vi "DAQ-AI Mean Value.vi"(8 "Cluster":T1, 11 "data":dbl[][](array[numeric]) format="%0.2f") -> (3 "Analoge Input":dbl[](array[numeric]))   [LabVIEW 2015]
uses:
  <vilib>/Analysis/baseanly.llb/Mean (DBL).vi
  Galobal variable_TI.vi
  <vilib>/Analysis/NI_AALBase.lvlib
  <vilib>/ptbypt/NI_PtbyPt.lvlib
panel:
  out "AI_as DI":bool[](array[boolean])
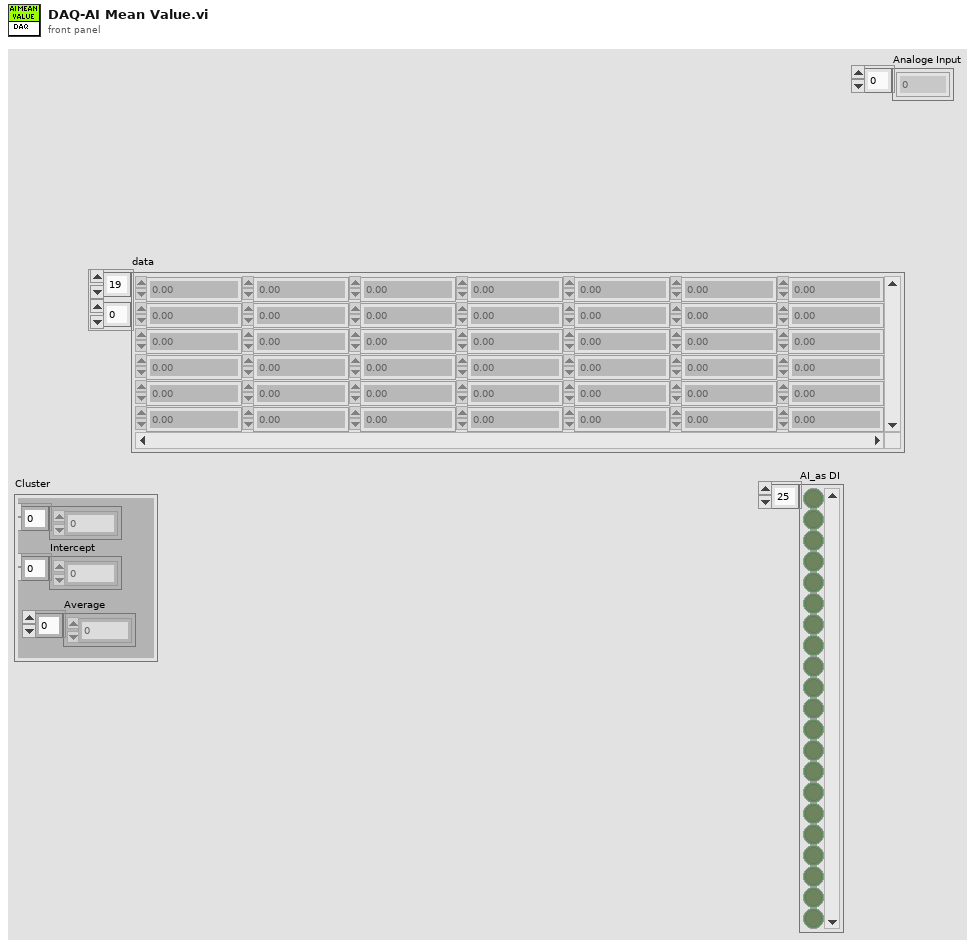
[diagram p1: front panel]
types:
  T1 = cluster{"Slop":dbl[], "Intercept":dbl[], "Average ":i16[]}
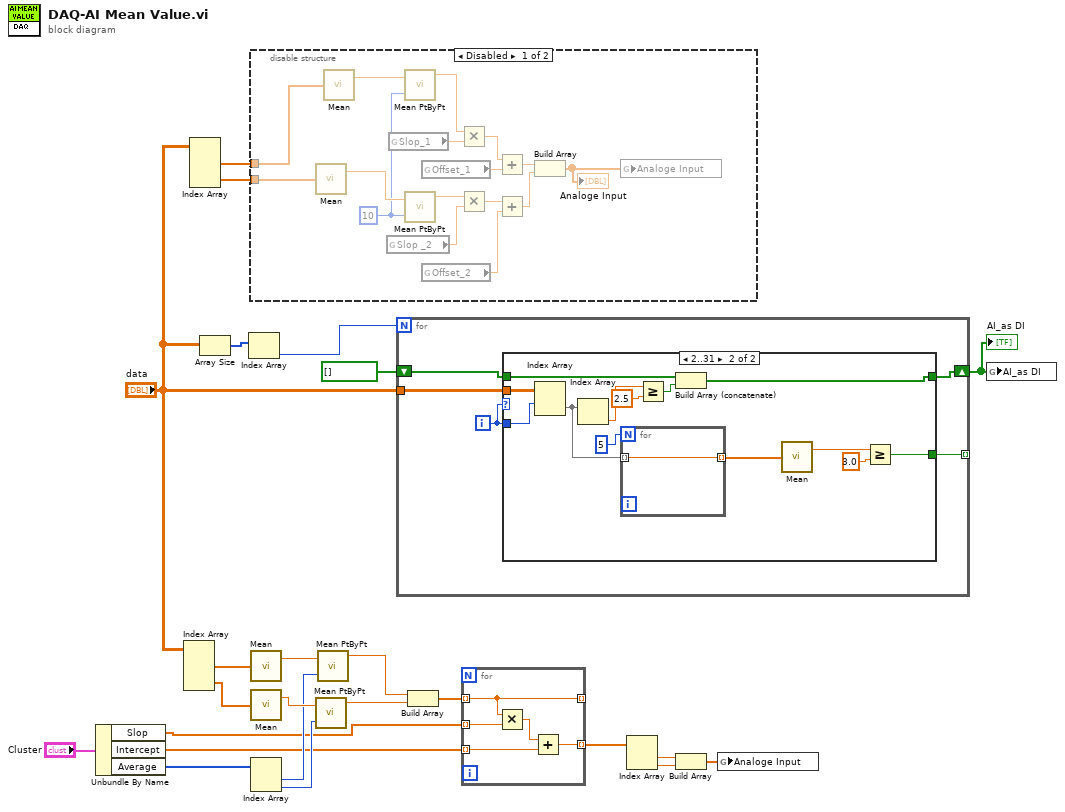
[diagram p0: block diagram]
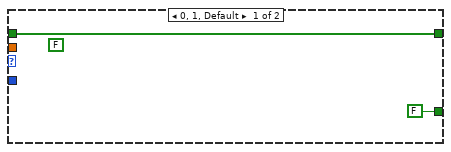
[diagram p3: hidden frame]
diagram:
  n1 = Unbundle By Name("Cluster") -> ("Slop"=w3:dbl[], "Intercept"=w2:dbl[], "Average"=w1:i16[])
  n2 = Index Array(array="data") -> (element #1=w9:dbl[], element #2=w8:dbl[])  [unwired: 4 in]
  n3 = Index Array(array="data") -> (element #1=w21:dbl[], element #2=w24:dbl[])  [unwired: 4 in]
  n4 = Array Size(array="data") -> (size(s)=w23:i32[])
  n5 = Index Array(array=w23) -> (element=w20:i32)  [unwired: 1 in]
  n6 = disable-structure shown="Disabled" {
    disable-tunnel: w24 -> [w40 _]
    disable-tunnel: w21 -> [w37 _]
    frame Disabled {
      w36 = 10 ("sample length")
      n7 = call-poly <vilib>:"Mean.vi"("X"=w40) -> ("mean"=w38:dbl)  [unwired: 1 out]
      n8 = call-poly <vilib>:"Mean.vi"("X"=w37) -> ("mean"=w39:dbl)  [unwired: 1 out]
      n9 = global read "Galobal variable_TI.vi" "Slop _2"() -> (w28:dbl)
      n10 = global read "Galobal variable_TI.vi" "Slop_1"() -> (w33:dbl)
      n11 = call <vilib>:"Mean PtByPt.vi"("x"=w39, "sample length"=w36) -> ("mean"=w34:dbl)  [unwired: 2 in, 1 out]
      n12 = call <vilib>:"Mean PtByPt.vi"("x"=w38, "sample length"=w36) -> ("mean"=w29:dbl)  [unwired: 2 in, 1 out]
      n13 = global read "Galobal variable_TI.vi" "Offset_1"() -> (w31:dbl)
      n14 = global read "Galobal variable_TI.vi" "Offset_2"() -> (w27:dbl)
      n15 = Multiply(x=w34, y=w33) -> (x*y=w32:dbl)
      n16 = Multiply(x=w29, y=w28) -> (x*y=w30:dbl)
      n17 = Add(x=w32, y=w31) -> (x+y=w26:dbl)
      n18 = Add(x=w30, y=w27) -> (x+y=w25:dbl)
      n19 = Build Array(w26, w25) -> (w35:dbl[])
      "Analoge Input" <- w35
      n20 = global write "Galobal variable_TI.vi" "Analoge Input"(w35) -> ()
    }
    frame Enabled {
    }
  }
  n21 = call-poly <vilib>:"Mean.vi"("X"=w9) -> ("mean"=w17:dbl)  [unwired: 1 out]
  n22 = call-poly <vilib>:"Mean.vi"("X"=w8) -> ("mean"=w16:dbl)  [unwired: 1 out]
  n23 = Index Array(array=w1) -> (element #1=w15:i16, element #2=w14:i16)  [unwired: 2 in]
  n24 = call <vilib>:"Mean PtByPt.vi"("x"=w16, "sample length"=w14) -> ("mean"=w10:dbl)  [unwired: 2 in, 1 out]
  n25 = call <vilib>:"Mean PtByPt.vi"("x"=w17, "sample length"=w15) -> ("mean"=w11:dbl)  [unwired: 2 in, 1 out]
  n26 = for {
    N: w20 -> [_]
    tunnel: "data" -> [w45]
    tunnel: [w44] -> _ mode=indexing
    shift-right: [w42] -> w19
    shift-left: bool[] [] -> [w41]
    i -> [w43]
    n27 = case shown="2..31" w43 {
      tunnel: w45 -> [_ w60]
      tunnel: w43 -> [_ w51]
      tunnel: [FALSE w52] -> w44
      tunnel: [w46 w49] -> w42
      tunnel: w41 -> [w46 w48]
      frame 0, 1, Default {
        (unwired) FALSE
      }
      frame 2..31 {
        n28 = Index Array(array=w60, index (row)=w51) -> (element=w57:dbl[])  [unwired: 1 in]
        n29 = Index Array(array=w57) -> (element=w59:dbl)  [unwired: 1 in]
        n30 = for {
          N: 5 -> [_]
          tunnel: w57 -> [w61] mode=indexing
          tunnel: [w61] -> w55 mode=indexing
        }
        n31 = Greater Or Equal?(x=w59, y=2.5) -> (x >= y?=w50:bool)
        n32 = Build Array (concatenate)(w48, w50) -> (w49:bool[])
        n33 = call-poly <vilib>:"Mean.vi"("X"=w55) -> ("mean"=w53:dbl)  [unwired: 1 out]
        n34 = Greater Or Equal?(x=w53, y=3.0) -> (x >= y?=w52:bool)
      }
    }
  }
  "AI_as DI" <- w19
  n35 = Build Array(w11, w10) -> (w12:dbl[])
  n36 = for {
    tunnel: w3 -> [w66] mode=indexing
    tunnel: w2 -> [w64] mode=indexing
    tunnel: w12 -> [w63] mode=indexing
    tunnel: [w63] -> _ mode=indexing
    tunnel: [w62] -> w13 mode=indexing
    n37 = Multiply(x=w63, y=w66) -> (x*y=w65:dbl)
    n38 = Add(x=w65, y=w64) -> (x+y=w62:dbl)
  }
  n39 = Index Array(array=w13) -> (element #1=w6:dbl, element #2=w5:dbl)  [unwired: 2 in]
  n40 = Build Array(w6, w5) -> (w4:dbl[])
  n41 = global write "Galobal variable_TI.vi" "Analoge Input"(w4) -> ()
  n42 = global write "Galobal variable_TI.vi" "AI_as DI"(w19) -> ()
